vi "Framework.Number of Transceiver Threads.vi"(8 "error in (no error)":errorcluster, 10 "transceiver count":i32, 11 "Framework in":refnum<class "Framework.lvclass">) -> (0 "error out":errorcluster, 3 "Framework out":refnum<class "Framework.lvclass">)   [LabVIEW 2017, in "DSF.Engine.lvlib" / "Framework.lvclass"]
uses:
  Framework.lvclass
  Framework.lvclass/Framework.ctl
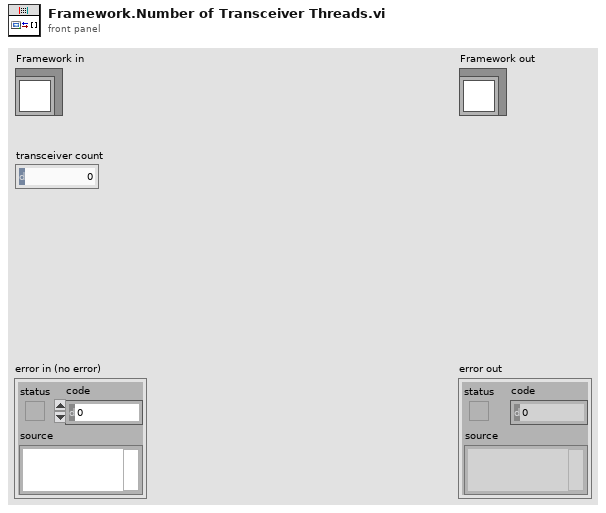
[diagram p1: front panel]
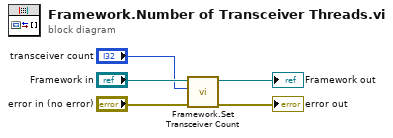
[diagram p0: block diagram]
diagram:
  n1 = call "Framework.Set Transceiver Count.vi"("transceiver count"="transceiver count", "Framework in"="Framework in") -> ("Framework out"=→"Framework out":refnum<class "Framework.lvclass">)  [unwired: 9 in]
  "error out" <- "error in (no error)"
